vi "DMM6500_Initialize_Msg_Queue_FGV.vi"(8 "error in (no error)":errorcluster, 11 "queue In":refnum<queue>) -> (0 "error out":errorcluster)   [LabVIEW 2024, in "DMM6500.lvlib"]
doc: "ThisVI\n---------------------------------\nInitialize_Queue_FGV\n---------------------------------\n-initialize the FGV Message Queue"
uses:
  DMM6500.lvlib
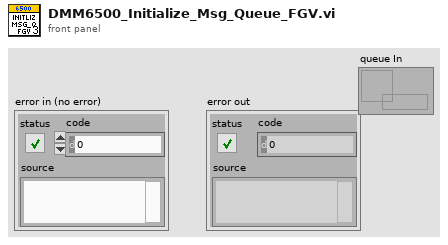
[diagram p1: front panel]
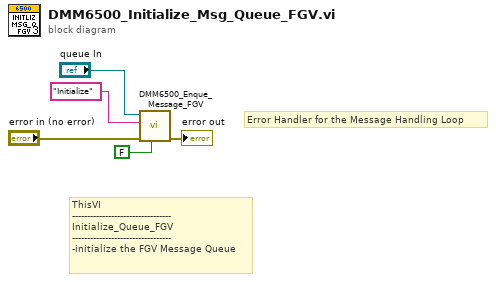
[diagram p0: block diagram]
diagram:
  # "Error Handler for the Message Handling Loop"
  # "ThisVI\n---------------------------------\nInitialize_Queue_FGV\n---------------------------------\n-initialize the FGV Message Queue"
  n1 = call "DMM6500_Enque_Message_FGV.vi"("Priority"=FALSE, "error in (no error)"="error in (no error)", "Message"="Initialize", "queue In"="queue In") -> ("error out"=→"error out":errorcluster)  [unwired: 7 in]
